vi "Tracking Test DAA.vi"(8 "error in (no error)":errorcluster, 10 "Model in":refnum<class "Model.lvclass">, 11 "Test Actuator State in":refnum<class "Test Actuator State.lvclass">) -> (0 "error out":errorcluster, 1 "Pass":bool, 2 "Model out":refnum<class "Model.lvclass">, 3 "Test Actuator State out":refnum<class "Test Actuator State.lvclass">)   [LabVIEW 2016]
uses:
  Model/Model/Model.lvclass
  Typedefs/ActuatorSetPoints.ctl
  <vilib>/Analysis/NI_AALPro.lvlib
  <vilib>/Analysis/5stat.llb/RMS (DBL).vi
  <vilib>/Analysis/NI_AALBase.lvlib
  <vilib>/Analysis/baseanly.llb/Mean (DBL).vi
  Model/Waveforms/Waveform/Waveform.lvclass
  <vilib>/platform/TimedLoop/XDataNode/XDataNode.xnode
  <vilib>/Platform/TimedLoop/XDataNode/nitl_modes.ctl
  <vilib>/Platform/TimedLoop/XDataNode/XDNodeRunTimeDep.lvlib
  <vilib>/Platform/TimedLoop/XDataNode/wakeup.ctl
  <vilib>/Platform/TimedLoop/XDataNode/timing_clust.ctl
  Test Actuator State.lvclass
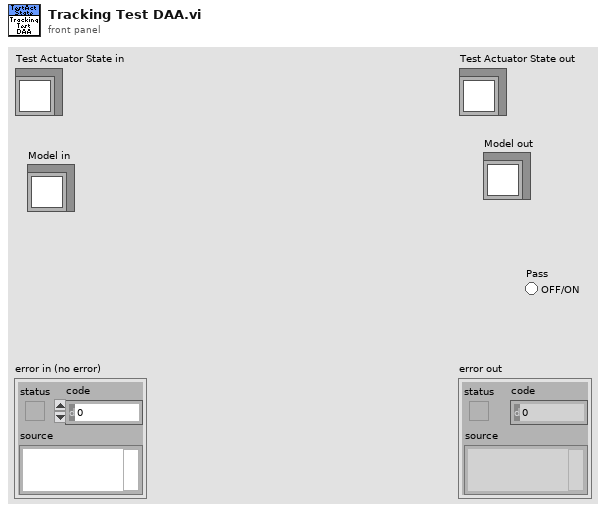
[diagram p1: front panel]
types:
  T1 = typedef "TrackingTestSettings.ctl" = cluster{"Max Force Error (N)":dbl, "Max Moment (NM)":dbl, "Process Time (s)":dbl, "Sample Time (s)":dbl, "Iterations":i32, "Amplitude (N)":dbl, "Non-Repeating Error":dbl}
  T2 = typedef "XDNodeRunTimeDep.lvlib/timing_clust.ctl" = cluster{"Expected End [f-1]":u64, "Actual End [f-1]":u64, "Finished Late? [f-1]":bool, "Expected End [i-1]":u64, "Actual End [i-1]":u64, "Finished Late? [i-1]":bool, "Expected Start [i]":u64, "Actual Start [i]":u64, "Expected Start [f]":u64, "Actual Start [f]":u64, "Source Name":string, "Structure Name":string, "Period":i64, "Deadline":i64, "Offset":i64, "Start":i64, "Priority":i32, "Timeout":i32, "Mode":T3, "Wakeup Reason":T4, "Error":errorcluster, "Source Type":string, "Secondary Source Type":string, "Global End Time":u64, "Global Start Time":u64, "Frame Duration":u64, "Iteration Duration":u64, "Assigned CPU":i32, "I/O Scan Engine Mode":u32}
  T3 = typedef "XDNodeRunTimeDep.lvlib/nitl_modes.ctl" = enum32{"No Change", "Process missed periods, maintain original phase", "Discard missed periods, maintain original phase", "Process missed periods, ignore original phase", "Discard missed periods, ignore original phase"}
  T4 = typedef "XDNodeRunTimeDep.lvlib/wakeup.ctl" = enum32{"Normal", "Aborted", "Asynchronous wakeup", "Timing source error", "Timed loop error", "Timeout"}
  T5 = typedef "ActuatorSetPoints.ctl" = cluster{"Axial Force":dbl, "Lateral Force":dbl, "FC1 Force":dbl, "FC2 Force":dbl}
  T6 = typedef "ActuatorData.ctl" = cluster{"Timestamp":dbl, "Force":dbl, "Encoder Value":i32}
  T7 = typedef "ToveyEngData.ctl" = cluster{"Timestamp":dbl, "Fx":dbl, "Fy":dbl, "Fz":dbl, "Mx":dbl, "My":dbl, "Mz":dbl}
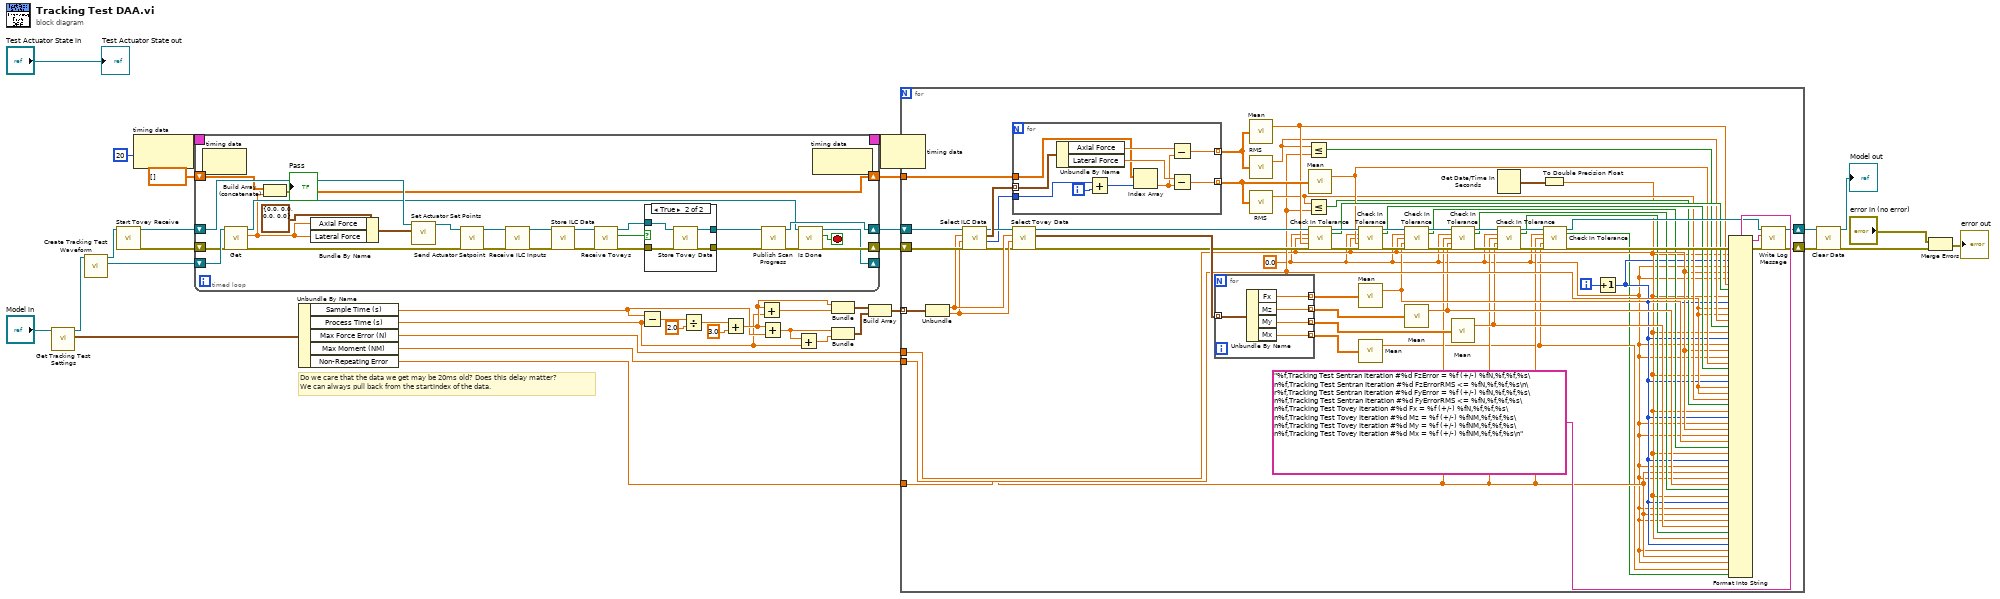
[diagram p0: block diagram]
diagram:
  # "Do we care that the data we get may be 20ms old? Does this delay matter?\nWe can always pull back from the startIndex of the data."
  n1 = call "Get Tracking Test Settings.vi"("Model in"="Model in") -> ("Tracking Test Settings"=w32:T1, "Model out"=w33:refnum<class "Model.lvclass">)  [unwired: 9 in]
  n2 = call "Create Tracking Test Waveform.vi"("Model in"=w33) -> ("Waveform"=w26:refnum<class "Waveform.lvclass">, "Model out"=w27:refnum<class "Model.lvclass">)  [unwired: 9 in]
  n3 = call "Start Tovey Receive.vi"("Model in"=w27) -> ("error out"=w28:errorcluster, "Model out"=w29:refnum<class "Model.lvclass">)  [unwired: 9 in]
  n4 = node-c288(i64 20 ("Period")) -> (w3:T2)
  n5 = timed-loop {
    shift-right: [w60] -> w25
    shift-left: w29 -> [w52]
    shift-right: [w43] -> w24
    shift-left: w28 -> [w46]
    shift-right: [w41] -> _
    shift-left: w26 -> [w48]
    shift-right: [w38] -> w4
    shift-left: dbl[] [] -> [w40]
    timing: w3 -> [_]
    timing-out: [_] -> w2
    stop <- w42 stop-if-true
    n6 = node-c288() -> ()  [unwired: 1 in, 1 out]
    n7 = call-dynamic "Get.vi"("error in (no error)"=w46, "Waveform in"=w48) -> ("error out"=w45:errorcluster, "Value"=w39:dbl, "Waveform out"=w47:refnum<class "Waveform.lvclass">)  [unwired: 7 in]
    n8 = Build Array (concatenate)(w40, w39) -> (w38:dbl[])
    n9 = Bundle By Name(cluster=T5 {"Axial Force"=0.0, "Lateral Force"=0.0, "FC1 Force"=0.0, "FC2 Force"=0.0} ("Actuator Set Points"), "Axial Force"=w39, "Lateral Force"=w39) -> (w49:T5)
    n10 = call "Set Actuator Set Points.vi"("Actuator Set Points"=w49, "Model in"=w52) -> ("Model out"=w51:refnum<class "Model.lvclass">)  [unwired: 9 in]
    n11 = call "Send Actuator Setpoint.vi"("error in (no error)"=w45, "Model in"=w51) -> ("error out"=w62:errorcluster, "Model out"=w64:refnum<class "Model.lvclass">)  [unwired: 8 in]
    n12 = call "Receive ILC Inputs.vi"("error in (no error)"=w62, "Model in"=w64) -> ("error out"=w61:errorcluster, "Model out"=w63:refnum<class "Model.lvclass">)  [unwired: 8 in]
    n13 = call "Store ILC Data.vi"("error in (no error)"=w61, "Model in"=w63) -> ("error out"=w58:errorcluster, "Model out"=w59:refnum<class "Model.lvclass">)  [unwired: 8 in]
    n14 = call "Receive Toveys.vi"("error in (no error)"=w58, "Model in"=w59) -> ("error out"=w56:errorcluster, "Data Received"=w55:bool, "Model out"=w57:refnum<class "Model.lvclass">)  [unwired: 7 in]
    n15 = case shown="True" w55 {
      tunnel: w57 -> [w68 w72]
      tunnel: w56 -> [w67 w71]
      tunnel: [w67 w70] -> w53
      tunnel: [w68 w69] -> w54
      frame False {
      }
      frame True {
        n16 = call "Store Tovey Data.vi"("error in (no error)"=w71, "Model in"=w72) -> ("error out"=w70:errorcluster, "Model out"=w69:refnum<class "Model.lvclass">)  [unwired: 8 in]
      }
    }
    n17 = call "Publish Scan Progress.vi"("error in (no error)"=w53, "Model in"=w54) -> ("error out"=w44:errorcluster, "Model out"=w60:refnum<class "Model.lvclass">)  [unwired: 8 in]
    n18 = call-dynamic "Is Done.vi"("error in (no error)"=w44, "Waveform in"=w47) -> ("error out"=w43:errorcluster, "Is Done"=w42:bool, "Waveform out"=w41:refnum<class "Waveform.lvclass">)  [unwired: 7 in]
    n19 = node-c288() -> ()  [unwired: 1 in, 1 out]
  }
  n20 = Unbundle By Name(w32) -> ("Sample Time (s)"=w14:dbl, "Process Time (s)"=w12:dbl, "Max Force Error (N)"=w23:dbl, "Max Moment (NM)"=w6:dbl, "Non-Repeating Error"=w7:dbl)
  n21 = Subtract(x=w14, y=w12) -> (x-y=w20:dbl)
  n22 = Divide(x=w20, y=2.0) -> (x/y=w18:dbl)
  n23 = Add(x=w18, y=3.0) -> (x+y=w15:dbl)
  n24 = Add(x=w15, y=w12) -> (x+y=w16:dbl)
  n25 = Add(x=w15, y=w14) -> (x+y=w13:dbl)
  n26 = Add(x=w13, y=w12) -> (x+y=w11:dbl)
  n27 = Bundle(w15, w16) -> (w10:cluster{dbl, dbl})  [unwired: 1 in]
  n28 = Bundle(w13, w11) -> (w9:cluster{dbl, dbl})  [unwired: 1 in]
  n29 = Build Array(w10, w9) -> (w8:cluster{dbl, dbl}[])
  n30 = node-c288(w2) -> ()  [unwired: 1 out]
  n31 = for {
    tunnel: w8 -> [w132] mode=indexing
    shift-right: [w116] -> w21
    shift-left: w25 -> [w131]
    shift-right: [w117] -> w22
    shift-left: w24 -> [w129]
    tunnel: w23 -> [w87]
    tunnel: w6 -> [w78]
    tunnel: w7 -> [w89]
    tunnel: w4 -> [w74]
    i -> [w121]
    w77 = 0.0
    n32 = Unbundle(w132) -> (w127:dbl, w126:dbl)
    n33 = call "Select ILC Data.vi"("error in (no error)"=w129, "End Time"=w126, "Start Time"=w127, "Model in"=w131) -> ("error out"=w125:errorcluster, "StartIndex"=w73:i32, "Data"=w130:T6[], "Model out"=w128:refnum<class "Model.lvclass">)  [unwired: 4 in]
    n34 = for {
      tunnel: w130 -> [w147] mode=indexing
      tunnel: [w145] -> w98 mode=indexing
      tunnel: [w143] -> w97 mode=indexing
      tunnel: w74 -> [w139]
      tunnel: w73 -> [w142]
      i -> [w141]
      n35 = Unbundle By Name(w147) -> ("Axial Force"=w146:dbl, "Lateral Force"=w144:dbl)
      n36 = Add(x=w142, y=w141) -> (x+y=w140:i32)
      n37 = Index Array(array=w139, index=w140) -> (element=w138:dbl)
      n38 = Subtract(x=w146, y=w138) -> (x-y=w145:dbl)
      n39 = Subtract(x=w144, y=w138) -> (x-y=w143:dbl)
    }
    n40 = call "Select Tovey Data.vi"("error in (no error)"=w125, "End Time"=w126, "Start Time"=w127, "Model in"=w128) -> ("error out"=w119:errorcluster, "Data"=w124:T7[], "Model out"=w120:refnum<class "Model.lvclass">)  [unwired: 4 in, 1 out]
    n41 = for {
      tunnel: [w137] -> w110 mode=indexing
      tunnel: [w136] -> w109 mode=indexing
      tunnel: [w135] -> w106 mode=indexing
      tunnel: [w134] -> w103 mode=indexing
      tunnel: w124 -> [w133] mode=indexing
      n42 = Unbundle By Name(w133) -> ("Fx"=w137:dbl, "Mz"=w136:dbl, "My"=w135:dbl, "Mx"=w134:dbl)
    }
    n43 = call-poly <vilib>:"Mean.vi"("X"=w98) -> ("mean"=w96:dbl)  [unwired: 1 out]
    n44 = call-poly <vilib>:"RMS.vi"("X"=w98) -> ("rms value"=w94:dbl)  [unwired: 1 out]
    n45 = call-poly <vilib>:"RMS.vi"("X"=w97) -> ("rms value"=w90:dbl)  [unwired: 1 out]
    n46 = Less Or Equal?(x=w94, y=w89) -> (x <= y?=w93:bool)
    n47 = Less Or Equal?(x=w90, y=w89) -> (x <= y?=w88:bool)
    n48 = call-poly <vilib>:"Mean.vi"("X"=w97) -> ("mean"=w92:dbl)  [unwired: 1 out]
    n49 = call "Check In Tolerance.vi"("Model in"=w120, "Expected"=w77, "Tolerance"=w87, "Actual"=w96, "error in (no error)"=w119) -> ("Model out"=w113:refnum<class "Model.lvclass">, "Pass"=w95:bool, "error out"=w114:errorcluster)  [unwired: 8 in]
    n50 = call "Check In Tolerance.vi"("Model in"=w113, "Expected"=w77, "Tolerance"=w87, "Actual"=w92, "error in (no error)"=w114) -> ("Model out"=w112:refnum<class "Model.lvclass">, "Pass"=w91:bool, "error out"=w111:errorcluster)  [unwired: 8 in]
    n51 = call-poly <vilib>:"Mean.vi"("X"=w110) -> ("mean"=w86:dbl)  [unwired: 1 out]
    n52 = call-poly <vilib>:"Mean.vi"("X"=w103) -> ("mean"=w76:dbl)  [unwired: 1 out]
    n53 = call "Check In Tolerance.vi"("Model in"=w112, "Expected"=w77, "Tolerance"=w87, "Actual"=w86, "error in (no error)"=w111) -> ("Model out"=w108:refnum<class "Model.lvclass">, "Pass"=w85:bool, "error out"=w107:errorcluster)  [unwired: 8 in]
    n54 = call-poly <vilib>:"Mean.vi"("X"=w109) -> ("mean"=w84:dbl)  [unwired: 1 out]
    n55 = call "Check In Tolerance.vi"("Model in"=w108, "Expected"=w77, "Tolerance"=w78, "Actual"=w84, "error in (no error)"=w107) -> ("Model out"=w105:refnum<class "Model.lvclass">, "Pass"=w83:bool, "error out"=w104:errorcluster)  [unwired: 8 in]
    n56 = call-poly <vilib>:"Mean.vi"("X"=w106) -> ("mean"=w82:dbl)  [unwired: 1 out]
    n57 = Get Date/Time In Seconds() -> (seconds since 1Jan1904=w122:timestamp)
    n58 = call "Check In Tolerance.vi"("Model in"=w105, "Expected"=w77, "Tolerance"=w78, "Actual"=w82, "error in (no error)"=w104) -> ("Model out"=w102:refnum<class "Model.lvclass">, "Pass"=w81:bool, "error out"=w100:errorcluster)  [unwired: 8 in]
    n59 = To Double Precision Float(number=w122) -> (double precision float=w80:dbl)
    n60 = call "Check In Tolerance.vi"("Model in"=w102, "Expected"=w77, "Tolerance"=w78, "Actual"=w76, "error in (no error)"=w100) -> ("Model out"=w101:refnum<class "Model.lvclass">, "Pass"=w75:bool, "error out"=w99:errorcluster)  [unwired: 8 in]
    n61 = Increment(x=w121) -> (x+1=w79:i32)
    n62 = Format Into String(format string="%f,Tracking Test Sentran Iteration #%d FzError = %f (+/-) %fN,%f,%f,%s\n%f,Tracking Test Sentran Iteration #%d FzErrorRMS <= %fN,%f,%f,%s\n\r%f,Tracking Test Sentran Iteration #%d FyError = %f (+/-) %fN,%f,%f,%s\n%f,Tracking Test Sentran Iteration #%d FyErrorRMS <= %fN,%f,%f,%s\n%f,Tracking Test Tovey Iteration #%d Fx = %f (+/-) %fN,%f,%f,%s\n%f,Tracking Test Tovey Iteration #%d Mz = %f (+/-) %fNM,%f,%f,%s\n%f,Tracking Test Tovey Iteration #%d My = %f (+/-) %fNM,%f,%f,%s\n%f,Tracking Test Tovey Iteration #%d Mx = %f (+/-) %fNM,%f,%f,%s\n", error in=w99, w80, w79, w77, w87, w77, w96, w95, w80, w79, w89, w89, w94, w93, w80, w79, w77, w87, w77, w92, w91, w80, w79, w89, w89, w90, w88, w80, w79, w77, w87, w77, w86, w85, w80, w79, w77, w78, w77, w84, w83, w80, w79, w77, w78, w77, w82, w81, w80, w79, w77, w78, w77, w76, w75) -> (resulting string=w115:string, error out=w118:errorcluster)  [unwired: 1 in]
    n63 = call "Write Log Message.vi"("error in (no error)"=w118, "Message"=w115, "Model in"=w101) -> ("error out"=w117:errorcluster, "Model out"=w116:refnum<class "Model.lvclass">)  [unwired: 7 in]
  }
  n64 = call "Clear Data.vi"("error in (no error)"=w22, "Model in"=w21) -> ("error out"=w31:errorcluster, "Model out"=→"Model out":refnum<class "Model.lvclass">)  [unwired: 8 in]
  n65 = Merge Errors("error in (no error)", w31) -> (→"error out":errorcluster)
  "Test Actuator State out" <- "Test Actuator State in"
